vi "Generate Relays.vi"() -> ()   [LabVIEW 2015]
uses:
  Classes/SLSC Switch/Controls/JSON.Relay.ctl
  Classes/SLSC Switch/Controls/JSON.RelaySLSCAction.ctl
panel:
  out "JSON string":string
  in  "relay":T1
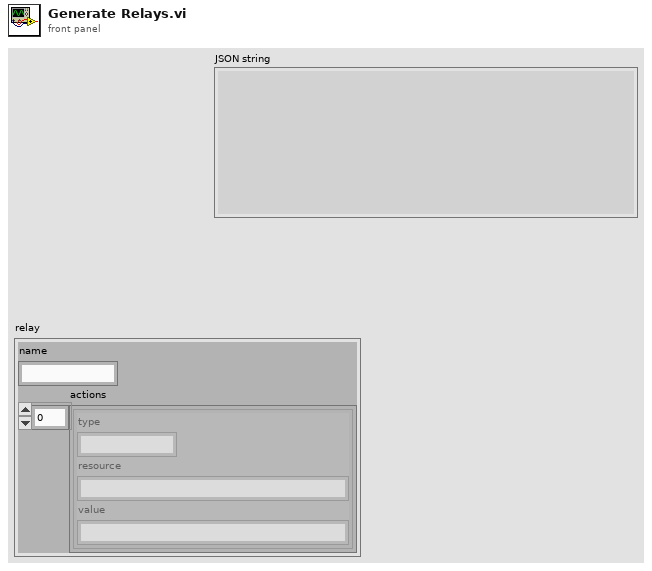
[diagram p1: front panel]
types:
  T1 = typedef "JSON.Relay.ctl" = cluster{"name":string, "actions":T2[]}
  T2 = typedef "JSON.RelaySLSCAction.ctl" = cluster{"type":string, "resource":string, "value":string}
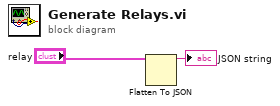
[diagram p0: block diagram]
diagram:
  n1 = Flatten To JSON(anything="relay") -> (JSON string=→"JSON string":string)  [unwired: 2 in, 1 out]
